vi "Section Names.vi"() -> (0 "Cluster":T1={"Conflict Zones"="Conflict Zones", "More Valves"="More Valves", "Pressure Display"="Pressure Display", "Temperature"="Temperature"})   [LabVIEW 2016, in "Hardware.lvlib" / "VacuumLine.lvlib" / "VacuumLines Configuration.lvclass"]
uses:
  <userlib>/Common Components/Hardware/Abstract System/VacuumLine/VacuumLines Configuration/VacuumLines Configuration.lvclass
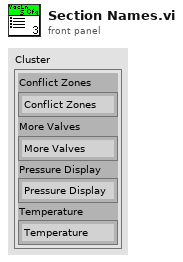
[diagram p1: front panel]
types:
  T1 = cluster{"Conflict Zones":string, "More Valves":string, "Pressure Display":string, "Temperature":string}
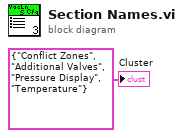
[diagram p0: block diagram]
diagram:
  "Cluster" <- T1 {"Conflict Zones"="Conflict Zones", "More Valves"="Additional Valves", "Pressure Display"="Pressure Display", "Temperature"="Temperature"} ("Cluster")
